vi "Write Working Path.vi"(11 "Working Path":path) -> ()   [LabVIEW 2020, in "SimpleDependencyInspector.lvlib"]
uses:
  <resource>/dialog/lvconfig.llb/LV Config Write Pathlist.vi
  SimpleDependencyInspector.lvlib
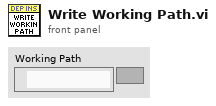
[diagram p1: front panel]
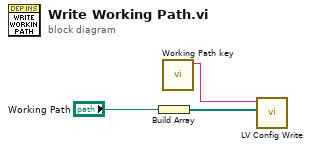
[diagram p0: block diagram]
diagram:
  n1 = Build Array("Working Path") -> (w3:path[])
  n2 = call "Working Path key.vi"() -> ("String"=w1:string)  [unwired: 11 in]
  n3 = call-poly <resource>:"LV Config Write.vi"("value"=w3, "key"=w1) -> ()  [unwired: 5 in, 1 out]
